vi "ReadMono.vi"(4 "Write Wait (10 ms)":u32, 5 "Busy":refnum<vi>, 6 "error in (no error)":errorcluster, 7 "Cmd":u16(ring) items=["?nm", "?nm/min", "?grating", "?turret", "?gratings"], 8 "Valid Read Time Out (10 sec)":dbl, 9 "Mono Port":refnum<visa-resource-name>) -> (0 "error out":errorcluster, 1 "Read Error":bool, 2 "Response":string, 3 "Mono Port Out":refnum<visa-resource-name>)   [LabVIEW 2009]
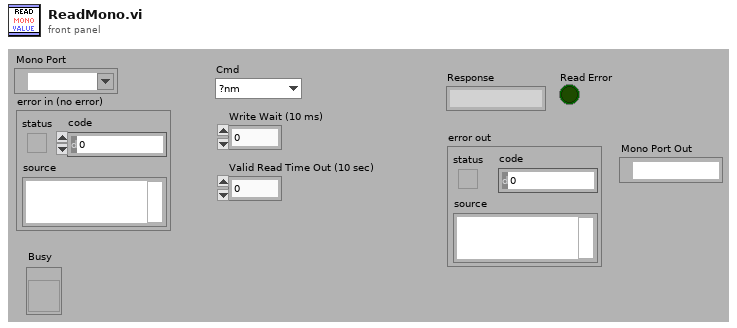
[diagram p1: front panel]
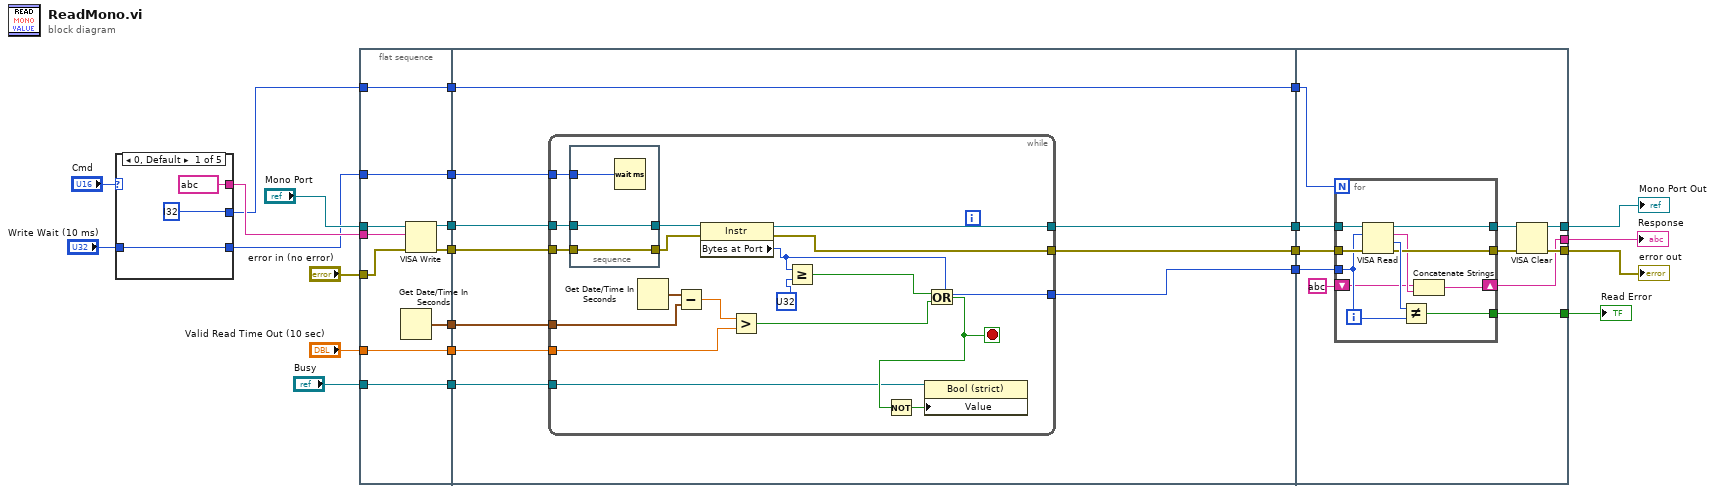
[diagram p0: block diagram]
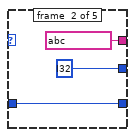
[diagram p2: hidden frame]
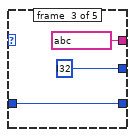
[diagram p3: hidden frame]
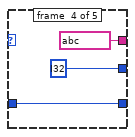
[diagram p4: hidden frame]
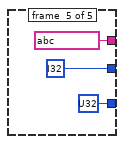
[diagram p5: hidden frame]
diagram:
  n1 = case shown="0, Default" "Cmd" {
    tunnel: [string ? string ? string ? string ? string ?] -> w21
    tunnel: [i32 ? ("y") i32 ? ("y") i32 ? ("y") i32 ? ("y") i32 ? ("y")] -> w8
    tunnel: [w25 w28 w31 w34 u32 ? ("Write Wait (5 ms)")] -> w4
    tunnel: "Write Wait (10 ms)" -> [w25 w28 w31 w34 _]
    frame #0 {
    }
    frame #1 {
    }
    frame #2 {
    }
    frame #3 {
    }
    frame #4 {
    }
  }
  n2 = flat-sequence {
    tunnel: "Mono Port" -> [w49]
    tunnel: "error in (no error)" -> [w48]
    tunnel: w21 -> [w47]
    tunnel: [w46] -> w20
    tunnel: [w45] -> w19
    tunnel: [w44] -> w18
    tunnel: "Valid Read Time Out (10 sec)" -> [w43]
    tunnel: [w43] -> w9
    tunnel: w8 -> [w42]
    tunnel: [w42] -> w6
    tunnel: w4 -> [w41]
    tunnel: [w41] -> w3
    tunnel: [w40] -> w2
    tunnel: "Busy" -> [w40]
    tunnel: w20 -> [w59]
    tunnel: w19 -> [w58]
    tunnel: w18 -> [w57]
    tunnel: [w56] -> w17
    tunnel: [w55] -> w16
    tunnel: [w54] -> w15
    tunnel: w9 -> [w53]
    tunnel: [w52] -> w7
    tunnel: w6 -> [w52]
    tunnel: w3 -> [w51]
    tunnel: w2 -> [w50]
    tunnel: w17 -> [w91]
    tunnel: w16 -> [w90]
    tunnel: [w84] -> w11
    tunnel: [w85] -> w13
    tunnel: [w83] -> w12
    tunnel: [w89] -> w14
    tunnel: w15 -> [w88]
    tunnel: w7 -> [w82]
    frame #0 {
      n3 = Get Date/Time In Seconds() -> (seconds since 1Jan1904=w46:timestamp)
      n4 = VISA Write(VISA resource name=w49, write buffer=w47, error in (no error)=w48) -> (VISA resource name out=w45:refnum<visa-resource-name>, error out=w44:errorcluster)  [unwired: 1 out]
    }
    frame #1 {
      n5 = while {
        tunnel: w59 -> [w75]
        tunnel: w58 -> [w72]
        tunnel: w57 -> [w73]
        tunnel: [w69] -> w56
        tunnel: [w68] -> w55
        tunnel: [w66] -> w54
        tunnel: w53 -> [w67]
        tunnel: w51 -> [w63]
        tunnel: w50 -> [w61]
        stop <- w62 stop-if-true
        n6 = stacked-sequence {
          tunnel: [w79] -> w70
          tunnel: w72 -> [w80]
          tunnel: [w80] -> w71
          tunnel: w73 -> [w79]
          tunnel: w63 -> [w78]
          frame #0 {
            n7 = Wait (ms)(milliseconds to wait=w78) -> ()  [unwired: 1 out]
          }
        }
        n8 = Get Date/Time In Seconds() -> (seconds since 1Jan1904=w77:timestamp)
        n9 = Subtract(x=w77, y=w75) -> (x-y=w76:dbl)
        n10 = property class="Instr"(reference=w71, error in=w70) -> (reference out=w69:refnum<visa-resource-name>, error out=w68:errorcluster, "Bytes at Port"=w66:u32)
        n11 = Greater?(x=w76, y=w67) -> (0:w74:bool)
        n12 = Greater Or Equal?(x=w66, y=u32 ?) -> (x >= y?=w64:bool)
        n13 = Or(x=w64, y=w74) -> (x .or. y?=w62:bool)
        n14 = Not(x=w62) -> (.not. x?=w60:bool)
        n15 = property class="Bool (strict)"(reference=w61, "Value"=w60) -> ()  [unwired: 1 in, 2 out]
      }
    }
    frame #2 {
      n16 = for {
        N: w82 -> [_]
        tunnel: w91 -> [w101]
        tunnel: w90 -> [w100]
        tunnel: [w98] -> w89
        tunnel: w88 -> [w97]
        tunnel: [w96] -> w87
        tunnel: [w95] -> w86
        shift-right: [w92] -> w83
        shift-left: string ? -> [w93]
        n17 = VISA Read(VISA resource name=w101, byte count=w97, error in (no error)=w100) -> (VISA resource name out=w96:refnum<visa-resource-name>, read buffer=w94:string, return count=w99:u32, error out=w95:errorcluster)
        n18 = Not Equal?(x=w99, y=w97) -> (x != y?=w98:bool)
        n19 = Concatenate Strings(w93, w94) -> (w92:string)
      }
      n20 = VISA Clear(VISA resource name=w87, error in (no error)=w86) -> (VISA resource name out=w84:refnum<visa-resource-name>, error out=w85:errorcluster)
    }
  }
  "Read Error" <- w14
  "error out" <- w13
  "Response" <- w12
  "Mono Port Out" <- w11
